vi "SGUI Set Complex String By Label.vi"   [LabVIEW 2013, in "varilib.lvlib"]
doc: "Sets complex number to string control references by its label (must be first registered by calling 'SGUI Register Controls')."
uses:
  varilib.lvlib
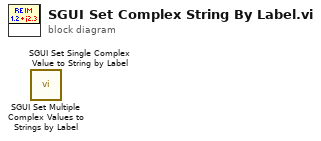
[diagram p0: block diagram]
diagram:
  n1 = call "SGUI Set Multiple Complex Values to Strings by Label.vi"() -> ()  [unwired: 14 in, 2 out]
  n2 = call "SGUI Set Single Complex Value to String by Label.vi"() -> ()  [unwired: 14 in, 2 out]
